vi "I_trial.vi"() -> ()   [LabVIEW 2023]
uses:
  Controls/Adresse.ctl
  TCxxxx.lvlib
panel:
  out "error out":errorcluster
  in  "flow control":u16(ring) items=["None"=0, "XON/XOFF"=1, "RTS/CTS"=2, "DTR/DSR"=4]
  in  "End write with termination character?":bool
  in  "Input\nbuffer size":u32=4096
  in  "Adresse 5":T1
  in  "Befehl \n[0 ... 65535] 4":u16
  in  "Parameter\n[0 ... 65535] 3":u16
  out "Regler Rückgabewert\n[0 ... 65535]":u16
  in  "write INT":bool
  in  "stop":bool
  in  "Adresse 4":T1
  in  "Befehl \n[0 ... 65535] 3":u16
  in  "Parameter \n[-32768 ... 0 ... 32767]":i16
  in  "Adresse 3":T1
  in  "Befehl \n[0 ... 65535] 2":u16
  in  "Parameter\n[0 ... 65535] 2":u16
  in  "write WORD":bool
  in  "read WORD":bool
  in  "Adresse 2":T1
  in  "Befehl \n[0 ... 65535]":u16
  in  "Parameter\n[0 ... 65535]":u16
  out "Regler Rückgabewert\n[-32768 ... 32767]":i16
  in  "read INT":bool
  in  "Adresse":T1
  in  "update":bool
  in  "termination char\n(0xA = '\\n' = LF)":u8=10 format="%.0x"
  in  "timeout (ms)":u32=10000
  in  "stop bits":u16(ring)=20 items=["1.0"=10, "1.5"=15, "2.0"=20]
  in  "parity":u16(ring) items=["None", "Odd", "Even", "Mark", "Space"]
  in  "data bits":u16=8 min=5 max=8 step=1
  in  "VISA resource name":refnum<visa-resource-name>="COM1"
  in  "baud rate":u32=9600
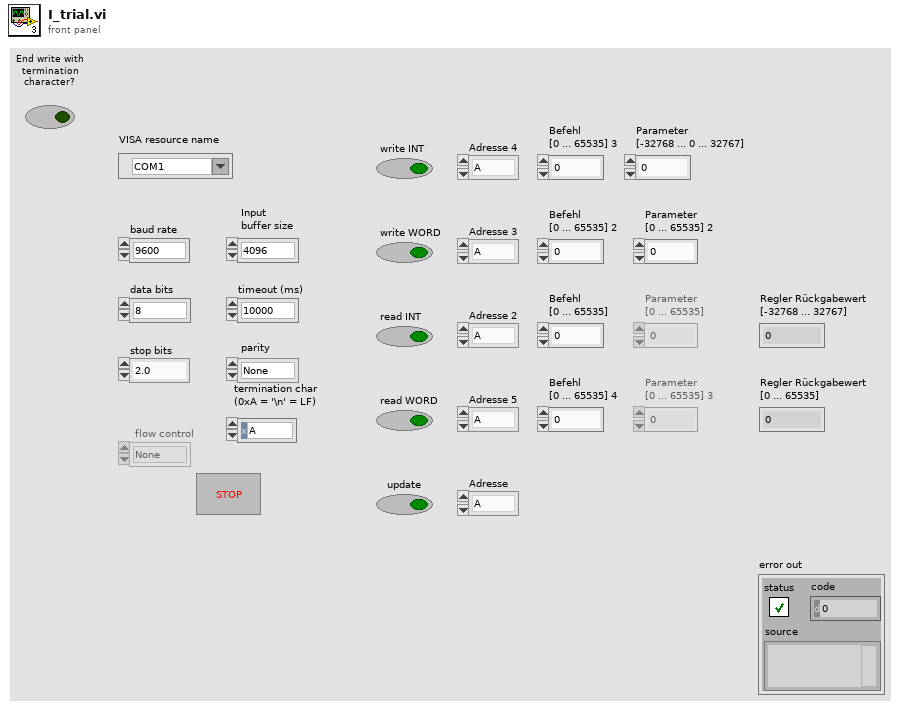
[diagram p1: front panel]
types:
  T1 = typedef "Adresse.ctl" = enum16{"A", "B", "C", "D", "E", "F", "G", "H", "I", "J", "K", "L", "M", "N", "O", "P", "Q", "R", "S", "T", "U", "V", "W", "X", "Y", "Z"}
  T2 = cluster{"Baud Rate":u32, "Parity":u16, "Data Bits":u16, "Stop Bits":u16, "Flow Control":u16}
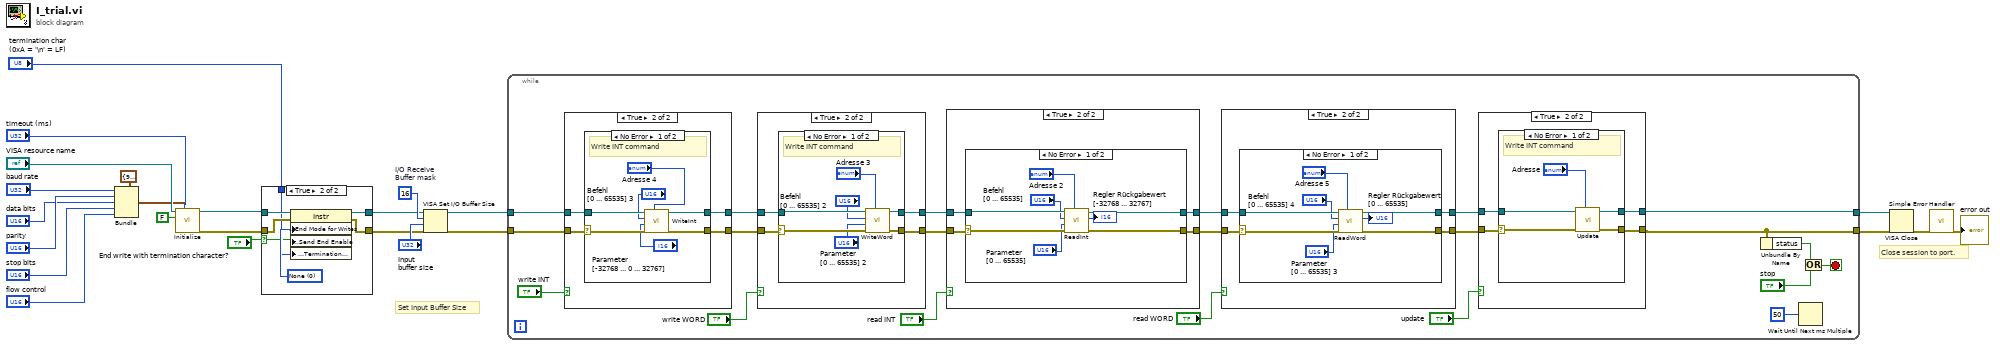
[diagram p0: block diagram]
diagram:
  w23 = u16 16  # I/O Receive Buffer mask
  # "Set Input Buffer Size"
  # "Close session to port."
  n1 = Bundle(cluster=T2 {"Baud Rate"=9600, "Parity"=0, "Data Bits"=8, "Stop Bits"=20, "Flow Control"=0} ("Serial Configuration"), "Baud Rate"="baud rate", "Parity"="parity", "Data Bits"="data bits", "Stop Bits"="stop bits", "Flow Control"="flow control") -> (w8:T2)
  n2 = call "Initialize.vi"("Timeout [ms]"="timeout (ms)", "Serial Configuration"=w8, "ID Query (True)"=FALSE, "VISA resource name"="VISA resource name") -> ("error out"=w5:errorcluster, "VISA resource name out"=w6:refnum<visa-resource-name>)  [unwired: 6 in]
  n3 = case shown="True" "End write with termination character?" {
    selector: "End write with termination character?" -> [_ w27]
    tunnel: w6 -> [w25 w33]
    tunnel: w5 -> [w26 w32]
    tunnel: [w25 w31] -> w18
    tunnel: [w26 w30] -> w19
    tunnel: "termination char\n(0xA = '\\n' = LF)" -> [_ w28]
    frame False {
    }
    frame True {
      w29 = u16 0 items=["None", "LastBit", "TermChar", "Break"] ("Serial Settings:Serial End Mode for Writes")
      n4 = property class="Instr"(reference=w33, error in=w32, "Serial Settings:End Mode for Writes"=w29, "Message Based Settings:Send End Enable"=w27, "Message Based Settings:Termination Character"=w28) -> (reference out=w31:refnum<visa-resource-name>, error out=w30:errorcluster)
    }
  }
  n5 = VISA Set I/O Buffer Size(VISA resource name=w18, mask (16)=w23, size (4096)="Input\nbuffer size", error in (no error)=w19) -> (VISA resource name out=w2:refnum<visa-resource-name>, error out=w1:errorcluster)
  n6 = while {
    tunnel: w1 -> [w50]
    tunnel: w2 -> [w51]
    tunnel: [w35] -> w17
    tunnel: [w36] -> w16
    stop <- w49 stop-if-true
    n7 = case shown="True" "write INT" {
      tunnel: [w100 w104] -> w47
      tunnel: [w99 w103] -> w45
      tunnel: w51 -> [w100 w102]
      tunnel: w50 -> [w99 w101]
      frame False {
      }
      frame True {
        n8 = case shown="No Error" w101 {
          selector: w101 -> [w110 w113]
          tunnel: [w108 w112] -> w104
          tunnel: [w109 w113] -> w103
          tunnel: w102 -> [w111 w112]
          frame No Error {
            # "Write INT command"
            n9 = call "WriteInt.vi"("Adresse"="Adresse 4", "error in (no error)"=w110, "Parameter [-32768 ... 0 ... 32767]"="Parameter \n[-32768 ... 0 ... 32767]", "Befehl [0 ... 65535]"="Befehl \n[0 ... 65535] 3", "VISA resource name"=w111) -> ("error out"=w109:errorcluster, "VISA resource name out"=w108:refnum<visa-resource-name>)  [unwired: 4 in, 1 out]
          }
          frame Error {
          }
        }
      }
    }
    n10 = case shown="True" "write WORD" {
      tunnel: [w85 w89] -> w43
      tunnel: [w84 w88] -> w42
      tunnel: w47 -> [w85 w87]
      tunnel: w45 -> [w84 w86]
      frame False {
      }
      frame True {
        n11 = case shown="No Error" w86 {
          selector: w86 -> [w96 w98]
          tunnel: [w90 w97] -> w89
          tunnel: [w91 w98] -> w88
          tunnel: w87 -> [w95 w97]
          frame No Error {
            # "Write INT command"
            n12 = call "WriteWord.vi"("Adresse"="Adresse 3", "error in (no error)"=w96, "Parameter [0 ... 65535]"="Parameter\n[0 ... 65535] 2", "Befehl [0 ... 65535]"="Befehl \n[0 ... 65535] 2", "VISA resource name"=w95) -> ("error out"=w91:errorcluster, "VISA resource name out"=w90:refnum<visa-resource-name>)  [unwired: 4 in, 1 out]
          }
          frame Error {
          }
        }
      }
    }
    n13 = case shown="True" "read INT" {
      tunnel: w42 -> [w68 w71]
      tunnel: w43 -> [w69 w70]
      tunnel: [w68 w73] -> w40
      tunnel: [w69 w72] -> w41
      frame False {
      }
      frame True {
        n14 = case "Read bytes from port." shown="No Error" w71 {
          selector: w71 -> [w80 w82]
          tunnel: [w79 w82] -> w73
          tunnel: [w78 w83] -> w72
          tunnel: w70 -> [w81 w83]
          frame No Error {
            n15 = call "ReadInt.vi"("Adresse"="Adresse 2", "error in (no error)"=w80, "Parameter [0 ... 65535]"="Parameter\n[0 ... 65535]", "Befehl [0 ... 65535]"="Befehl \n[0 ... 65535]", "VISA resource name"=w81) -> ("error out"=w79:errorcluster, "Regler Rückgabewert [-32768 ... 32767]"=→"Regler Rückgabewert\n[-32768 ... 32767]":i16, "VISA resource name out"=w78:refnum<visa-resource-name>)  [unwired: 3 in, 1 out]
          }
          frame Error {
            # "Error occurred \nreading Bytes at \nSerial Port"
          }
        }
      }
    }
    n16 = case shown="True" "read WORD" {
      tunnel: w40 -> [w114 w118]
      tunnel: w41 -> [w115 w117]
      tunnel: [w114 w116] -> w37
      tunnel: [w115 w119] -> w38
      frame False {
      }
      frame True {
        n17 = case "Read bytes from port." shown="No Error" w118 {
          selector: w118 -> [w126 w128]
          tunnel: [w124 w128] -> w116
          tunnel: [w125 w129] -> w119
          tunnel: w117 -> [w127 w129]
          frame No Error {
            n18 = call "ReadWord.vi"("Adresse"="Adresse 5", "error in (no error)"=w126, "Parameter [0 ... 65535]"="Parameter\n[0 ... 65535] 3", "Befehl [0 ... 65535]"="Befehl \n[0 ... 65535] 4", "VISA resource name"=w127) -> ("error out"=w124:errorcluster, "Regler Rückgabewert [0 ... 65535]"=→"Regler Rückgabewert\n[0 ... 65535]":u16, "VISA resource name out"=w125:refnum<visa-resource-name>)  [unwired: 3 in, 1 out]
          }
          frame Error {
            # "Error occurred \nreading Bytes at \nSerial Port"
          }
        }
      }
    }
    n19 = case shown="True" "update" {
      tunnel: [w56 w60] -> w35
      tunnel: [w55 w59] -> w36
      tunnel: w38 -> [w56 w58]
      tunnel: w37 -> [w55 w57]
      frame False {
      }
      frame True {
        n20 = case shown="No Error" w57 {
          selector: w57 -> [w64 w67]
          tunnel: [w63 w66] -> w60
          tunnel: [w62 w67] -> w59
          tunnel: w58 -> [w65 w66]
          frame No Error {
            # "Write INT command"
            n21 = call "Update.vi"("Adresse"="Adresse", "error in (no error)"=w64, "VISA resource name"=w65) -> ("error out"=w62:errorcluster, "VISA resource name out"=w63:refnum<visa-resource-name>)  [unwired: 7 in]
          }
          frame Error {
          }
        }
      }
    }
    n22 = Unbundle By Name(w36) -> ("status"=w53:bool)
    n23 = Wait Until Next ms Multiple(millisecond multiple=u32 50) -> ()  [unwired: 1 out]
    n24 = Or(x=w53, y="stop") -> (x .or. y?=w49:bool)
  }
  n25 = VISA Close(VISA resource name=w17, error in (no error)=w16) -> (error out=w24:errorcluster)
  n26 = call <vilib>:"Simple Error Handler.vi"("error in (no error)"=w24) -> ("error out"=→"error out":errorcluster)  [unwired: 1 in, 7 out]
